vi "GUNSC_toUnsc.vi"(3 "responseQ":string, 4 "ms timeout (-1)":i32=-1, 5 "key":string, 6 "bpp":i32, 7 "location 2":u64, 8 "error in (no error)":errorcluster, 9 "ele Read":u32, 10 "location":u64, 11 "command":string) -> (0 "error out":errorcluster, 1 "response":errorcluster)   [LabVIEW 2016]
panel:
  in  "command strct":T1
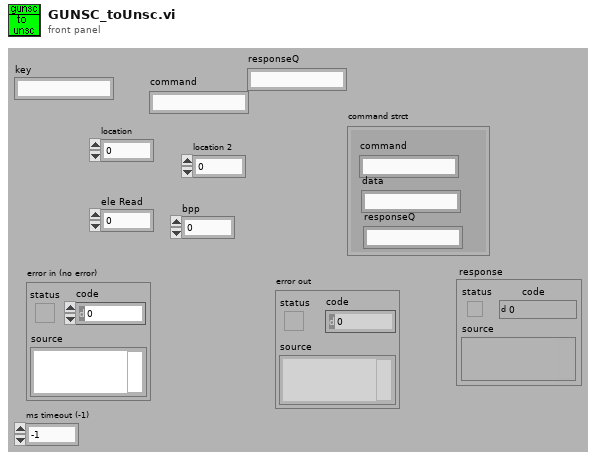
[diagram p1: front panel]
types:
  T1 = cluster{"command":string, "data":string, "responseQ":string}
  T2 = cluster{"location":u64, "ele Read":u32, "location 2":u64, "bpp":i32}
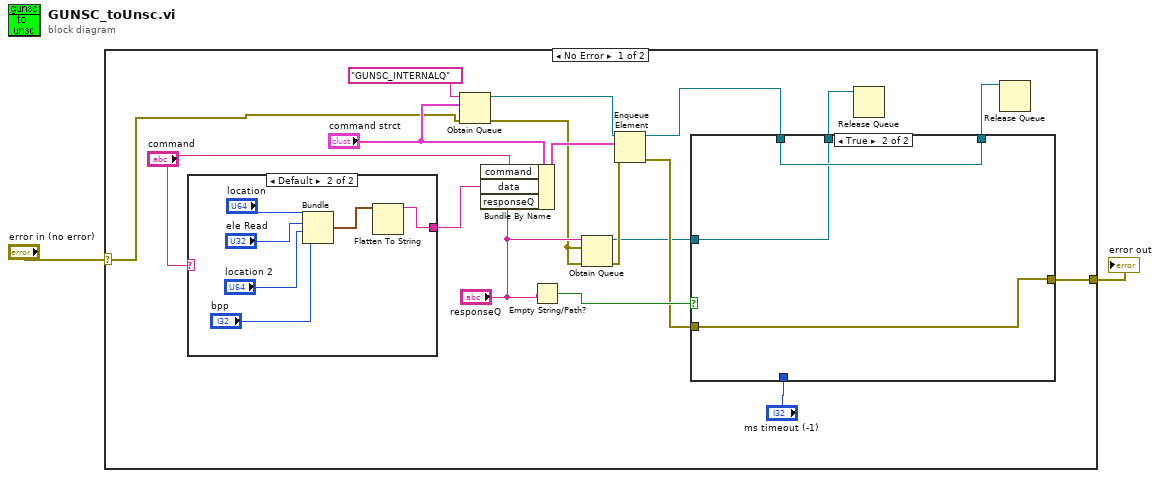
[diagram p0: block diagram]
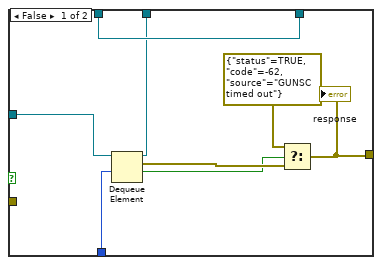
[diagram p2: hidden frame]
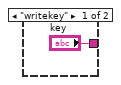
[diagram p3: hidden frame]
diagram:
  n1 = case shown="No Error" "error in (no error)" {
    selector: "error in (no error)" -> [w11 w39]
    tunnel: [w16 w39] -> w1
    frame No Error {
      n2 = case shown="Default" "command" {
        tunnel: ["key" w35] -> w20
        frame "writekey" {
        }
        frame Default {
          n3 = Bundle("location"="location", "ele Read"="ele Read", "location 2"="location 2", "bpp"="bpp") -> (w36:T2)  [unwired: 1 out]
          n4 = Flatten To String(anything=w36) -> (data string=w35:string)  [unwired: 1 in, 4 out]
        }
      }
      n5 = Obtain Queue(name (unnamed)="GUNSC_INTERNALQ", element data type="command strct", error in (no error)=w11) -> (queue out=w13:refnum<queue>, error out=w7:errorcluster)  [unwired: 2 in, 1 out]
      n6 = Bundle By Name(cluster="command strct", "command"="command", "data"=w20, "responseQ"="responseQ") -> (w12:T1)
      n7 = Empty String/Path?(string/path="responseQ") -> (empty?=w18:bool)
      n8 = Obtain Queue(name (unnamed)="responseQ", element data type=w7, error in (no error)=w7) -> (queue out=w4:refnum<queue>, error out=w6:errorcluster)  [unwired: 2 in, 1 out]
      n9 = Enqueue Element(queue=w13, element=w12, error in (no error)=w6) -> (queue out=w10:refnum<queue>, error out=w5:errorcluster)  [unwired: 2 out]
      n10 = case shown="True" w18 {
        tunnel: "ms timeout (-1)" -> [w26 _]
        tunnel: w5 -> [_ w31]
        tunnel: [w27 w31] -> w16
        tunnel: w10 -> [w23 w30]
        tunnel: [w23 w30] -> w9
        tunnel: w4 -> [w22 w29]
        tunnel: [w21 w29] -> w3
        frame False {
          n11 = Dequeue Element(queue=w22, timeout in ms (-1)=w26) -> (queue out=w21:refnum<queue>, element=w25:errorcluster, timed out?=w24:bool)  [unwired: 1 in, 1 out]
          n12 = Select(t=errorcluster {"status"=TRUE, "code"=-62, "source"="GUNSC timed out"}, s=w24, f=w25) -> (s? t:f=w27:errorcluster)
          "response" <- w27
        }
        frame True {
        }
      }
      n13 = Release Queue(queue=w3) -> ()  [unwired: 1 in, 4 out]
      n14 = Release Queue(queue=w9) -> ()  [unwired: 1 in, 4 out]
    }
    frame Error {
    }
  }
  "error out" <- w1
